vi "DPF.vi"(8 "errorIn":errorcluster, 11 "xmlFilePath":path) -> (0 "error out":errorcluster caption="errorOut", 3 "DPF":T1)   [LabVIEW 2017]
uses:
  models/DPF.ctl
  models/Header.ctl
  models/DPF_ocpeo.ctl
  models/DPF_operationMode.ctl
  models/DPF_command.ctl
  models/DPF_pidController.ctl
  models/DPF_engineLimit.ctl
  models/DPF_other.ctl
  <vilib>/xml/Load XML File.vi
  <vilib>/xml/NI_XML.lvlib
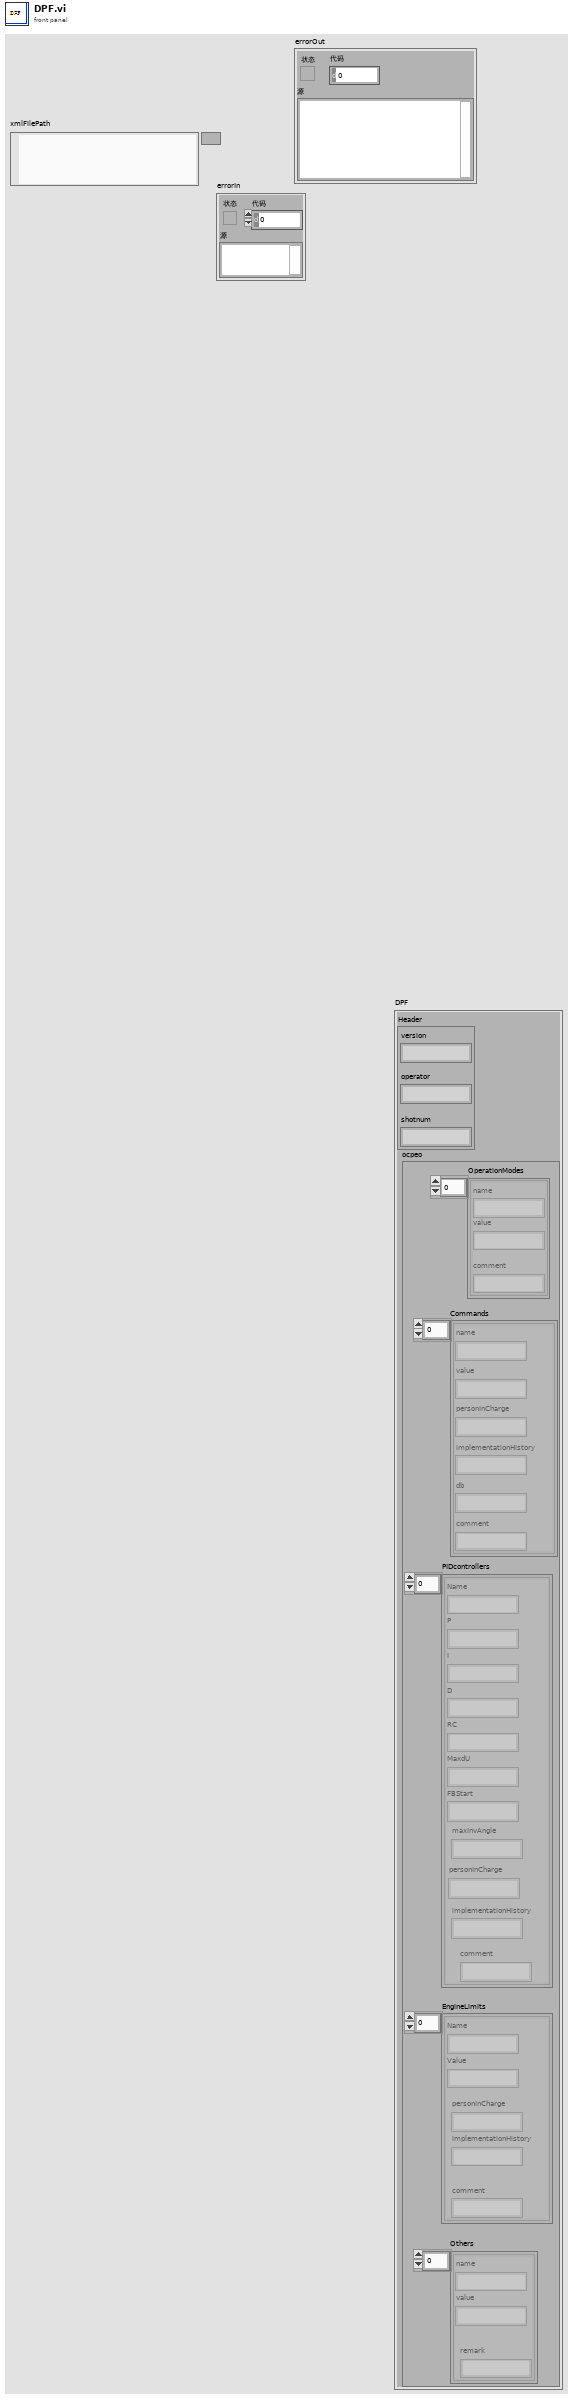
[diagram p1: front panel]
types:
  T1 = typedef "DPF.ctl" = cluster{"Header":T2, "ocpeo":T3}
  T2 = typedef "Header.ctl" = cluster{"version":string, "operator":string, "shotnum":string}
  T3 = typedef "DPF_ocpeo.ctl" = cluster{"OperationModes":T4[], "Commands":T5[], "PIDcontrollers":T6[], "EngineLimits":T7[], "Others":T8[]}
  T4 = typedef "DPF_operationMode.ctl" = cluster{"name":string, "value":string, "comment":string}
  T5 = typedef "DPF_command.ctl" = cluster{"name":string, "value":string, "personInCharge":string, "implementationHistory":string, "db":string, "comment":string}
  T6 = typedef "DPF_pidController.ctl" = cluster{"Name":string, "P":string, "I":string, "D":string, "RC":string, "MaxdU":string, "FBStart":string, "maxInvAngle":string, "personInCharge":string, "implementationHistory":string, "comment":string}
  T7 = typedef "DPF_engineLimit.ctl" = cluster{"Name":string, "Value":string, "personInCharge":string, "implementationHistory":string, "comment":string}
  T8 = typedef "DPF_other.ctl" = cluster{"name":string, "value":string, "remark":string}
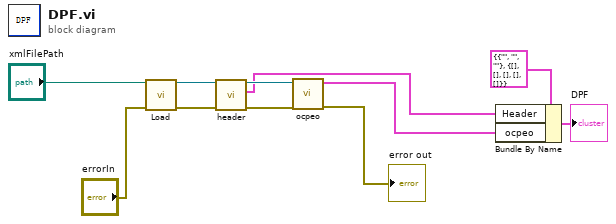
[diagram p0: block diagram]
diagram:
  n1 = call-poly <vilib>:"Load.vi"("path to XML document"="xmlFilePath", "error in (no error)"="errorIn") -> ("DOM document out"=w9:refnum<k20>, "error out"=w5:errorcluster)  [unwired: 11 in, 1 out]
  n2 = call "header.vi"("errorIn"=w5, "xmlRef"=w9) -> ("errorOut"=w10:errorcluster, "header"=w2:T2, "xmlRef"=w11:refnum<k20>)  [unwired: 7 in]
  n3 = call "ocpeo.vi"("error in"=w10, "xmlRef"=w11) -> ("error out"=→"error out":errorcluster, "ocpeo"=w3:T3)  [unwired: 8 in]
  n4 = Bundle By Name(cluster=T1 {"Header"={"version"="", "operator"="", "shotnum"=""}, "ocpeo"={"OperationModes"=[], "Commands"=[], "PIDcontrollers"=[], "EngineLimits"=[], "Others"=[]}} ("输入簇"), "Header"=w2, "ocpeo"=w3) -> (→"DPF":T1)
